vi "DmgrGetDvc.vi"(8 "Error In":errorcluster, 10 "Device Number":i32, 11 "Device Handle":u64) -> (0 "Error Out":errorcluster, 1 "Connection String":string, 2 "Name":string, 3 "Device Handle":u64, 4 "DTP":u32)   [LabVIEW 2011, in "LVH-Adept.lvlib" / "DMGR.lvlib"]
doc: "Get Device Handle"
uses:
  DMGR.lvlib
  Private/Type Defs/Error.ctl
  <vilib>/Utility/importsl/GetValueByPointer/datatype.ctl
  <vilib>/Utility/importsl/GetValueByPointer/GetValueByPointer.xnode
  Resources/dmgr.dll
  Program Files (x86)/National Instruments/LabVIEW 2011/resource/lvimptsl.dll
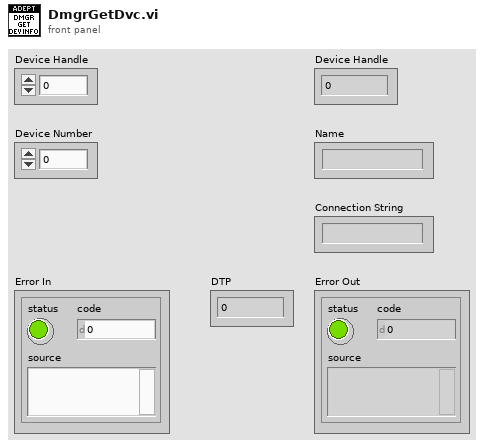
[diagram p1: front panel]
types:
  T1 = typedef "LVH-Adept.lvlib/DMGR.lvlib/Error.ctl" = enum16{"Unknown Error", "Device Enumeration", "Device Handle", "Device Info", "Device Open"}
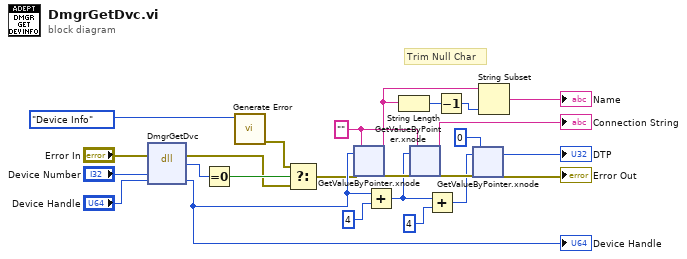
[diagram p0: block diagram]
diagram:
  w9 = ""
  # "Trim Null Char"
  n1 = dll-call lib="C:/github/makerhub/Adept/LabVIEW/vi.lib/MakerHub/Adept/Private/Resources/dmgr.dll" fn="DmgrGetDvc"(error in="Error In", "Device Number"="Device Number", "deviceHandlePtr"="Device Handle") -> (error out=w20:errorcluster, "Success"=w24:u8, "deviceHandlePtr"=w8:u64)  [unwired: 3 in, 1 out]
  "Device Handle" <- w8
  n2 = Equal To 0?(x=w24) -> (x = 0?=w23:bool)
  n3 = call "Generate Error.vi"("Error Type"=Error."Device Info") -> ("Error Out"=w21:errorcluster)  [unwired: 10 in]
  n4 = Select(t=w21, s=w23, f=w20) -> (s? t:f=w6:errorcluster)
  n5 = xnode "GetValueByPointer.xnode"("Pointer"=w8, "InputType"=w9, "ErrorIn"=w6) -> ("Output"=w3:string, "ErrorOut"=w17:errorcluster)  [unwired: 1 in]
  n6 = Add(x=w8, y=u64 4) -> (x+y=w13:u64)
  n7 = String Length(string=w3) -> (length=w2:i32)
  n8 = xnode "GetValueByPointer.xnode"("Pointer"=w13, "InputType"=w9, "ErrorIn"=w17) -> ("Output"=→"Connection String":string, "ErrorOut"=w16:errorcluster)  [unwired: 1 in]
  n9 = Add(x=w13, y=u64 4) -> (x+y=w12:u64)
  n10 = Decrement(x=w2) -> (x-1=w1:i32)
  n11 = xnode "GetValueByPointer.xnode"("Pointer"=w12, "InputType"=u32 0 ("y"), "ErrorIn"=w16) -> ("Output"=→"DTP":u32, "ErrorOut"=→"Error Out":errorcluster)  [unwired: 1 in]
  n12 = String Subset(string=w3, length (rest)=w1) -> (substring=→"Name":string)  [unwired: 1 in]
